vi "instantiate class.vi"() -> (4 "Espresso":refnum<class "Espresso.lvclass">, 15 "error out":errorcluster)   [LabVIEW 2021, in "Espresso.lvclass"]
uses:
  Espresso.lvclass
  Espresso.lvclass/Espresso.ctl
panel:
  # "Connector Pane"
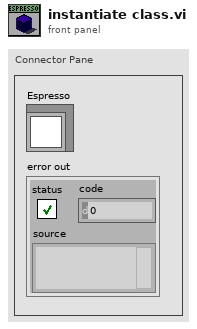
[diagram p1: front panel]
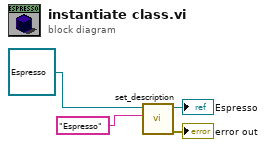
[diagram p0: block diagram]
diagram:
  n1 = call-dynamic "set_description.vi"("description"="Espresso", "object in"=refnum<class "Espresso.lvclass"> refnum ("Espresso.lvclass")) -> ("error out"=→"error out":errorcluster, "object out"=→"Espresso":refnum<class "Espresso.lvclass">)  [unwired: 8 in]
